vi "tabcouleur0.vi"(0 "Blue":string[](array[string]), 1 "Red":string[](array[string]), 2 "White":string[](array[string]), 3 "Green":string[](array[string]), 4 "Orange":string[](array[string]), 6 "Yellow":string[](array[string])) -> (7 "RubixTab solver":string[][](array[string]))   [LabVIEW 2019]
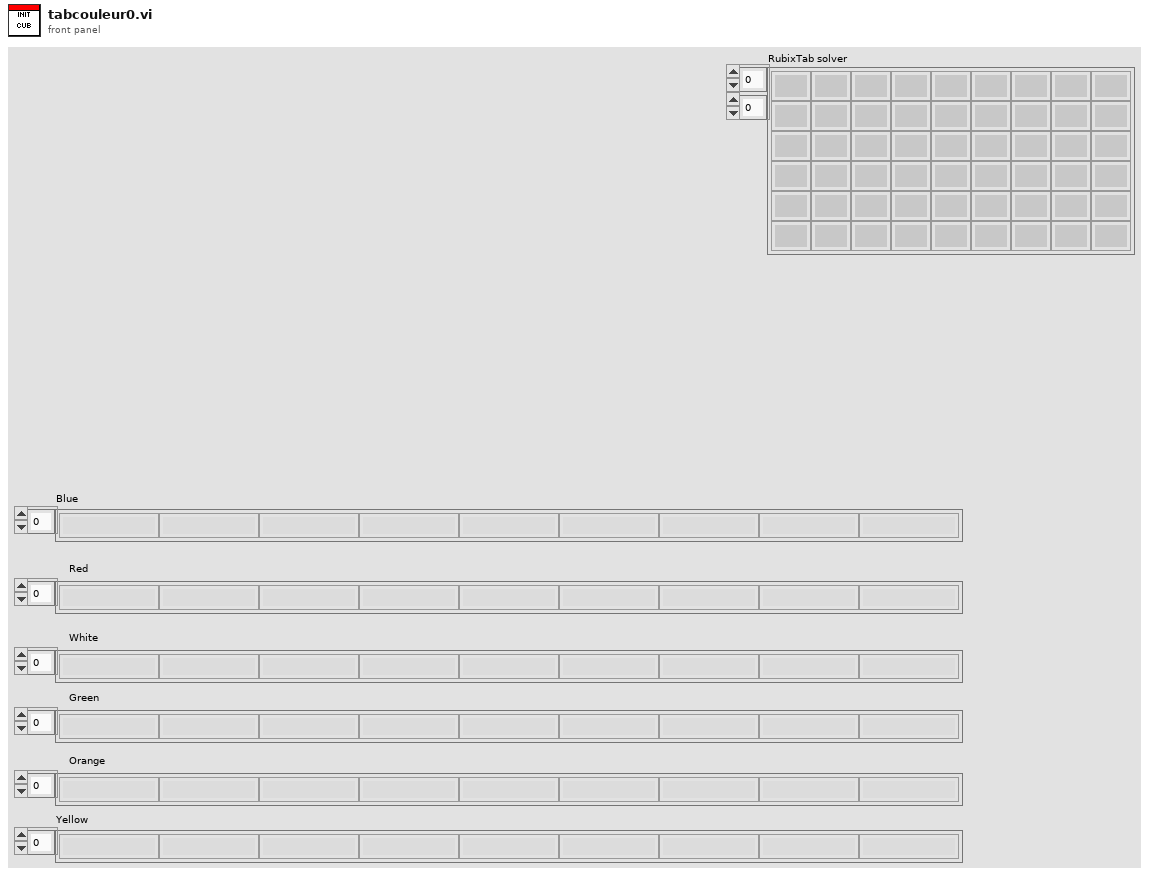
[diagram p1: front panel]
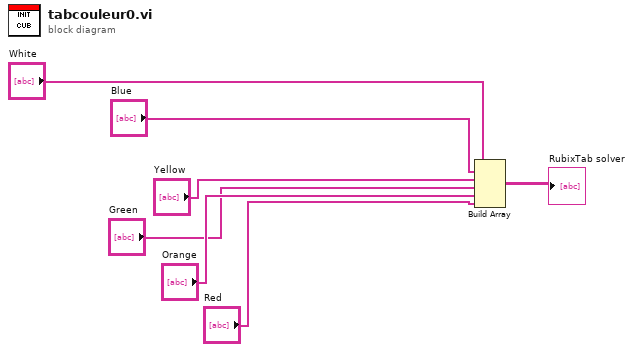
[diagram p0: block diagram]
diagram:
  n1 = Build Array("White", "Blue", "Yellow", "Green", "Orange", "Red") -> (→"RubixTab solver":string[][])
